vi "TeamDashDataCluster.vi"() -> ()   [LabVIEW 2011]
panel:
  in  "Team Dashboard Data":T1
  in  "Angle Trim":dbl
  in  "Velocity Trim":dbl
  in  "Locked":bool
  in  "Selected Target":dbl
  in  "Joystick Control":bool
  in  "Ball Count":dbl
  in  "Hopper Full":bool
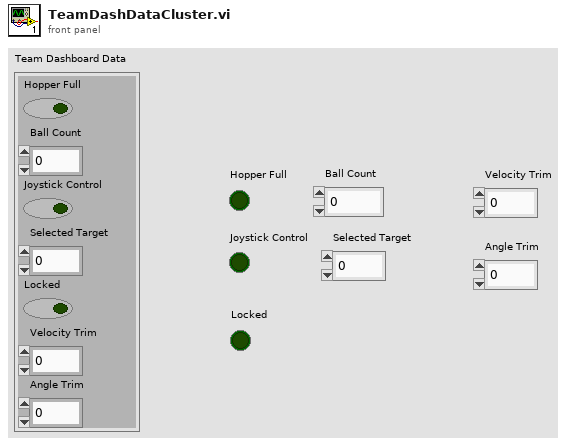
[diagram p1: front panel]
types:
  T1 = cluster{"Hopper Full":bool, "Ball Count":dbl, "Joystick Control":bool, "Selected Target":dbl, "Locked":bool, "Velocity Trim":dbl, "Angle Trim":dbl}
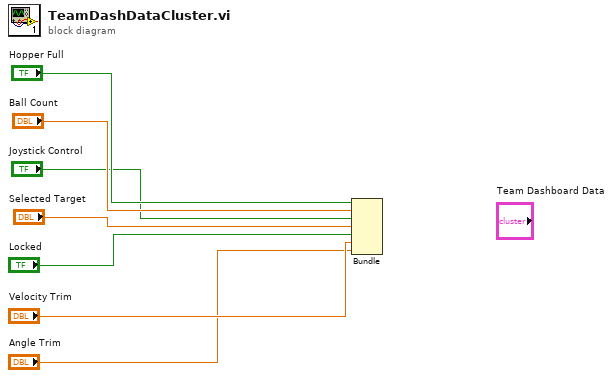
[diagram p0: block diagram]
diagram:
  n1 = Bundle("Hopper Full"="Hopper Full", "Ball Count"="Ball Count", "Joystick Control"="Joystick Control", "Selected Target"="Selected Target", "Locked"="Locked", "Velocity Trim"="Velocity Trim", "Angle Trim"="Angle Trim") -> ()  [unwired: 1 in, 1 out]
